vi "Create.vi"(10 "Path":path) -> (3 "PathValue out":refnum<class "PathValue.lvclass">)   [LabVIEW 2020, in "Volatus.lvlib" / "PathValue.lvclass"]
uses:
  PathValue.lvclass
  PathValue.lvclass/PathValue.ctl
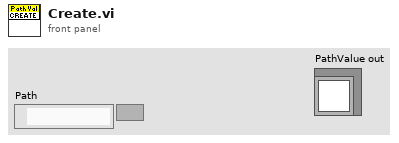
[diagram p1: front panel]
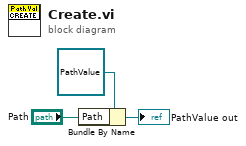
[diagram p0: block diagram]
diagram:
  n1 = Bundle By Name(cluster=refnum<class "PathValue.lvclass"> refnum ("PathValue in"), "Path"="Path") -> (→"PathValue out":refnum<class "PathValue.lvclass">)
